vi "UploadFirmware.vi"(1 "Firmware data":string[](array[string]), 2 "Devices":T1[](array[typedef])) -> (0 "Devices":T1[](array[typedef]))   [LabVIEW 2010]
uses:
  Controls/Device.ctl
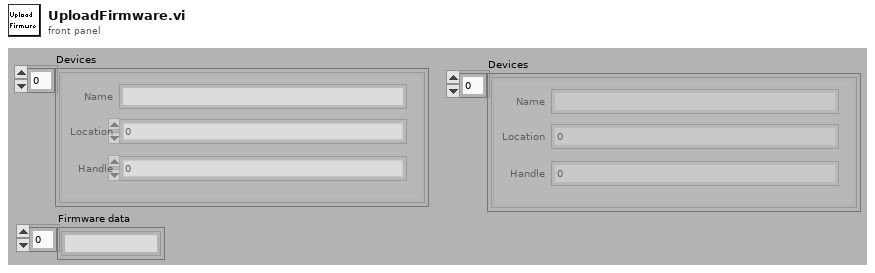
[diagram p1: front panel]
types:
  T1 = typedef "Device.ctl" = cluster{"Name":string, "Location":u32, "Handle":u32}
  T2 = cluster{"WaitDataWriteComplete":bool, "WaitDataWritePin":u32, "DataWriteCompleteState":bool, "DataWriteTimeoutmSecs":u32}
  T3 = cluster{"Clock Pin High":bool, "Data Out High":bool, "Chip Select High":bool, "Chip Select Pin":u32}
  T4 = cluster{"ClockOutDataBitsMSBFirst":bool, "ClockOutDataBitsPosEdge":bool, "NumControlBitsToWrite":u32, "WriteControlBuffer":u8[], "NumControlBytesToWrite":u32, "WriteDataBits":bool, "NumDataBitsToWrite":u32, "WriteDataBuffer":u8[], "NumDataBytesToWrite":u32}
  T5 = cluster{"GPIOH1 (ACBUS0) Active":bool, "GPIOH1 (ACBUS0) High":bool, "GPIOH2 (ACBUS1) Active":bool, "GPIOH2 (ACBUS1) High":bool, "GPIOH3 (ACBUS2) Active":bool, "GPIOH3 (ACBUS2) High":bool, "GPIOH4 (ACBUS3) Active":bool, "GPIOH4 (ACBUS3) High":bool}
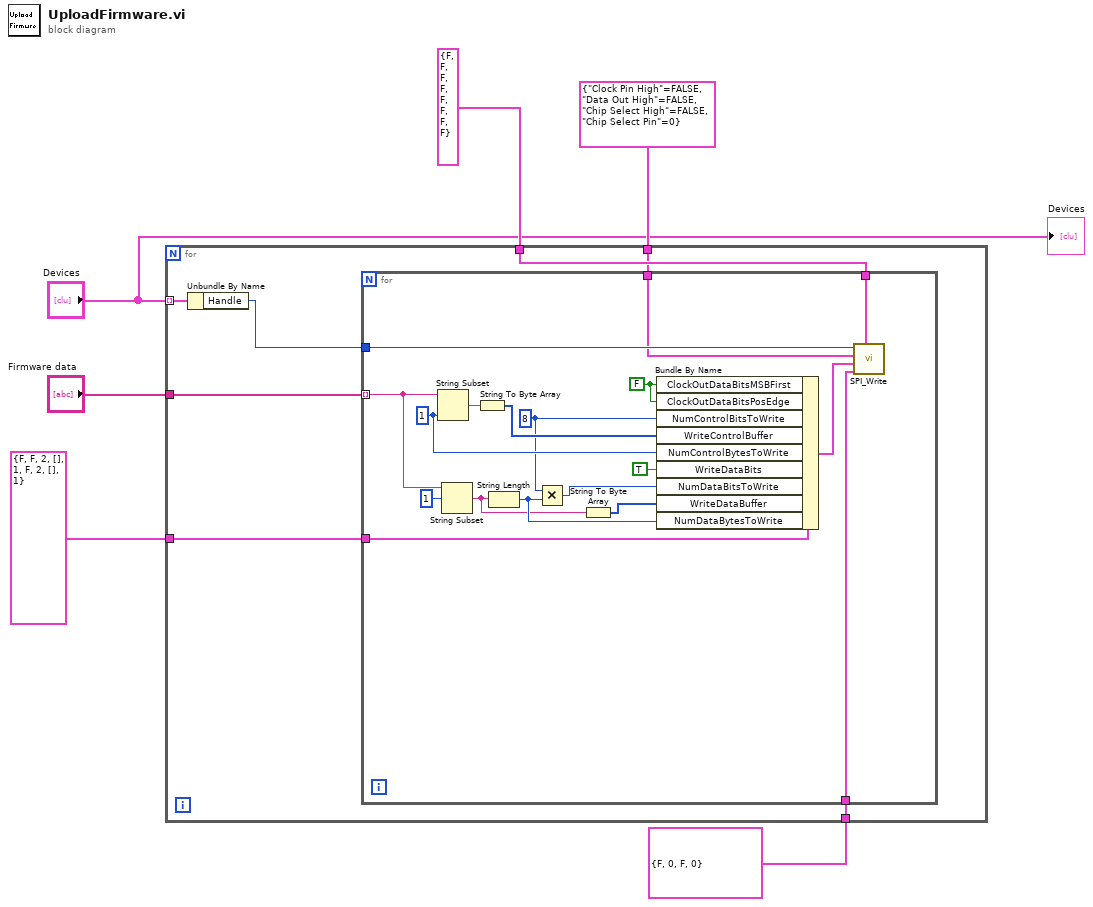
[diagram p0: block diagram]
diagram:
  n1 = for {
    tunnel: "Devices" -> [w12] mode=indexing
    tunnel: "Firmware data" -> [w13]
    tunnel: T5 {"GPIOH1 (ACBUS0) Active"=FALSE, "GPIOH1 (ACBUS0) High"=FALSE, "GPIOH2 (ACBUS1) Active"=FALSE, "GPIOH2 (ACBUS1) High"=FALSE, "GPIOH3 (ACBUS2) Active"=FALSE, "GPIOH3 (ACBUS2) High"=FALSE, "GPIOH4 (ACBUS3) Active"=FALSE, "GPIOH4 (ACBUS3) High"=FALSE} ("HighPinsWriteActiveStates") -> [w10]
    tunnel: T4 {"ClockOutDataBitsMSBFirst"=FALSE, "ClockOutDataBitsPosEdge"=FALSE, "NumControlBitsToWrite"=2, "WriteControlBuffer"=[], "NumControlBytesToWrite"=1, "WriteDataBits"=FALSE, "NumDataBitsToWrite"=2, "WriteDataBuffer"=[], "NumDataBytesToWrite"=1} ("Control and Data Bits") -> [w9]
    tunnel: T3 {"Clock Pin High"=FALSE, "Data Out High"=FALSE, "Chip Select High"=FALSE, "Chip Select Pin"=0} ("WriteStartCondition") -> [w8]
    tunnel: T2 {"WaitDataWriteComplete"=FALSE, "WaitDataWritePin"=0, "DataWriteCompleteState"=FALSE, "DataWriteTimeoutmSecs"=0} ("WaitDataWriteComplete") -> [w7]
    n2 = Unbundle By Name(w12) -> ("Handle"=w11:u32)
    n3 = for {
      tunnel: w13 -> [w22] mode=indexing
      tunnel: w11 -> [w31]
      tunnel: w10 -> [w30]
      tunnel: w9 -> [w29]
      tunnel: w8 -> [w15]
      tunnel: w7 -> [w14]
      w24 = 1 ("length (rest)")
      w20 = u32 8 ("NumControlBitsToWrite")
      w27 = FALSE ("ClockOutDataBitsMSBFirst")
      n4 = String Subset(string=w22, length (rest)=w24) -> (substring=w26:string)  [unwired: 1 in]
      n5 = String Subset(string=w22, offset (0)=1) -> (substring=w17:string)  [unwired: 1 in]
      n6 = String To Byte Array(string=w26) -> (unsigned byte array=w25:u8[])
      n7 = String Length(string=w17) -> (length=w19:i32)
      n8 = Multiply(x=w20, y=w19) -> (x*y=w18:u32)
      n9 = String To Byte Array(string=w17) -> (unsigned byte array=w16:u8[])
      n10 = Bundle By Name(cluster=w29, "ClockOutDataBitsMSBFirst"=w27, "ClockOutDataBitsPosEdge"=w27, "NumControlBitsToWrite"=w20, "WriteControlBuffer"=w25, "NumControlBytesToWrite"=w24, "WriteDataBits"=TRUE, "NumDataBitsToWrite"=w18, "WriteDataBuffer"=w16, "NumDataBytesToWrite"=w19) -> (w28:T4)
      n11 = call "SPI_Write.vi"("Handle"=w31, "WriteStartCondition"=w15, "Control and Data Bits"=w28, "WaitDataWriteComplete"=w14, "HighPinsWriteActiveStates"=w30) -> ()  [unwired: 1 out]
    }
  }
  "Devices" <- "Devices"
